vi "XYStage.KIM101.Close Device.vi"(8 "error in (no error)":errorcluster, 10 "Device":refnum<k24>, 11 "KCubeInertialMotorControl in":refnum<k24>) -> (0 "error out":errorcluster)   [LabVIEW 2017, in "XYStage.KIM101.lvclass"]
uses:
  XYStage.KIM101.lvclass
  C:/Program Files (x86)/Thorlabs/Kinesis/Thorlabs.MotionControl.Controls.dll
  C:/Program Files (x86)/Thorlabs/Kinesis/Thorlabs.MotionControl.KCube.InertialMotorCLI.dll
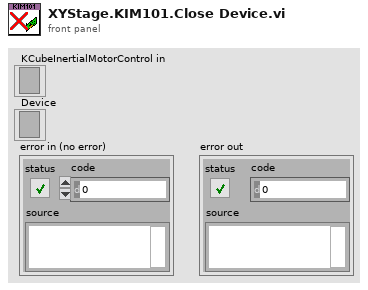
[diagram p1: front panel]
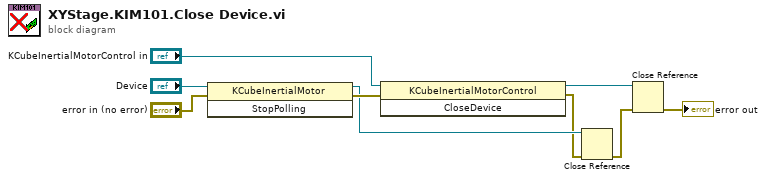
[diagram p0: block diagram]
diagram:
  n1 = invoke class="KCubeInertialMotor" method="StopPolling"(reference="Device", error in="error in (no error)") -> (reference out=w5:refnum<k24>, error out=w8:errorcluster)  [unwired: 1 in, 1 out]
  n2 = invoke class="KCubeInertialMotorControl" method="CloseDevice"(reference="KCubeInertialMotorControl in", error in=w8) -> (reference out=w4:refnum<k24>, error out=w3:errorcluster)  [unwired: 1 in, 1 out]
  n3 = Close Reference(reference=w5, error in (no error)=w3) -> (error out=w2:errorcluster)
  n4 = Close Reference(reference=w4, error in (no error)=w2) -> (error out=→"error out":errorcluster)
